vi "FastWriter.vi"() -> ()   [LabVIEW 2012]
uses:
  WVD-MCSupdate/WVDNewArchitectureUpdate/WVD_Architecture_Update/TypeDefinitions.llb/TypeDef_MPDUnitID.ctl
panel:
  out "Receive Buffer Size":u32
  out "WriteCount":i32
  out "LoopCount":i32
  out "error out":errorcluster
  in  "stop":bool
  in  "MPDUnitID":T1=enum."MPD#01"
  in  "DataBasePath":string="C:\\Users\\h2odial\\WVD-MCSupdate\\WVDNewArchitectureUpdate\\WVD_Architecture_Update\\Data\\TCSPC\\"
  in  "FileBaseNameIn":string="TCSPCFastData"
  in  "UDP Port":u16=54002
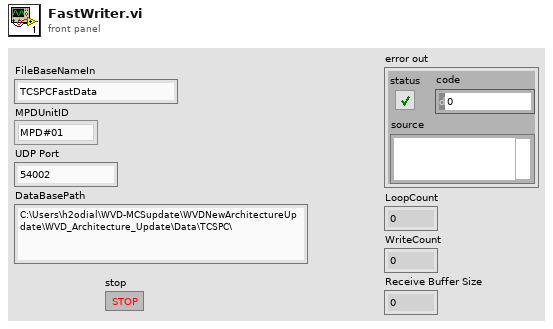
[diagram p1: front panel]
types:
  T1 = typedef "TypeDef_MPDUnitID.ctl" = enum8{"Unknown", "MPD#01", "MPD#02", "MPD#03", "MPD#04", "MPD#05"}
  T2 = enum16{"open", "replace", "create", "open or create", "replace or create", "replace or create with confirmation"}
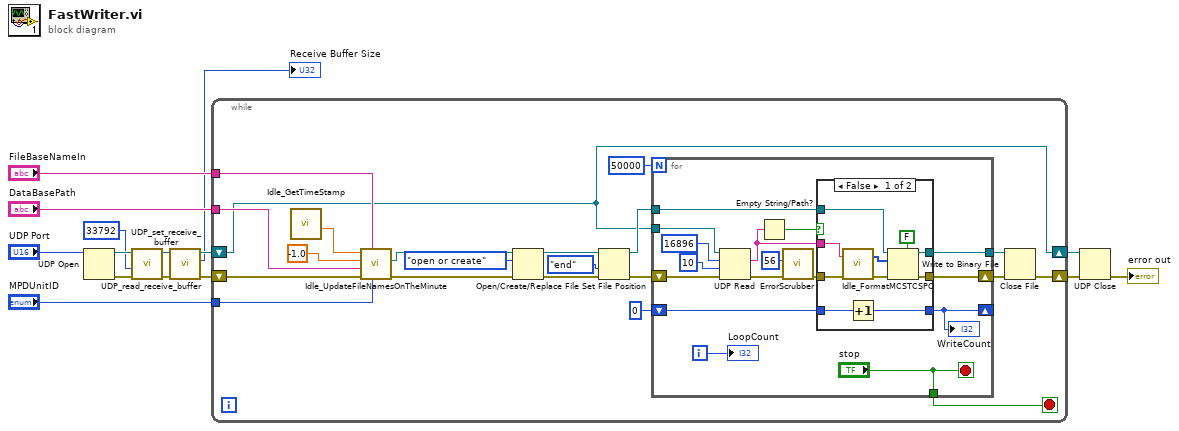
[diagram p0: block diagram]
diagram:
  n1 = UDP Open(11:"UDP Port") -> (port=w12:refnum<k16>, 0:w13:errorcluster)  [unwired: 4 in, 1 out]
  n2 = call "UDP_set_receive_buffer.vi"("error in (no error)"=w13, "Receive Buffer Size"=u32 33792, "connection ID"=w12) -> ("error out"=w10:errorcluster, "connection ID out"=w9:refnum<k16>)  [unwired: 6 in]
  n3 = call "UDP_read_receive_buffer.vi"("error in (no error)"=w10, "connection ID"=w9) -> ("error out"=w7:errorcluster, "Receive Buffer Size"=→"Receive Buffer Size":u32, "connection ID out"=w3:refnum<k16>)  [unwired: 5 in]
  n4 = while {
    shift-right: [w24] -> w15
    shift-left: w7 -> [w23]
    tunnel: "FileBaseNameIn" -> [w22]
    tunnel: "DataBasePath" -> [w21]
    tunnel: "MPDUnitID" -> [w20]
    shift-right: [w18] -> w2
    shift-left: w3 -> [w18]
    stop <- w19 stop-if-true
    n5 = call "Idle_GetTimeStamp.vi"() -> ("Fractional Hours"=w36:dbl)  [unwired: 11 in]
    n6 = call "Idle_UpdateFileNamesOnTheMinute.vi"("MPDUnitID"=w20, "FileBaseNameIn"=w22, "ErrorIn"=w23, "DataBasePathIn"=w21, "FileUpdateTimeIn"=-1.0, "CurrentTime"=w36) -> ("ErrorOur"=w30:errorcluster, "WritePathOut"=w29:path)  [unwired: 2 in, 2 out]
    n7 = Open/Create/Replace File(file path (use dialog)=w29, error in=w30, operation (0:open)=T2."open or create") -> (refnum out=w32:refnum<file>, error out=w31:errorcluster)  [unwired: 3 in, 1 out]
    n8 = Set File Position(refnum=w32, from (0:start)=enum16{"start", "end", "current"}."end", error in=w31) -> (refnum out=w28:refnum<file>, error out=w17:errorcluster)  [unwired: 1 in]
    n9 = for {
      N: 50000 -> [_]
      tunnel: w28 -> [w45]
      shift-right: [w43] -> _
      shift-left: 0 -> [w44]
      shift-right: [w41] -> w26
      shift-left: w17 -> [w42]
      tunnel: [w40] -> w25
      tunnel: w18 -> [w39]
      tunnel: ["stop"] -> w19
      i -> [w38]
      stop <- "stop" stop-if-true
      n10 = UDP Read(connection ID=w39, max size (548)=16896, timeout ms (25000)=10, 8:w42) -> (data out=w49:string, error out=w51:errorcluster)  [unwired: 3 out]
      n11 = Empty String/Path?(string/path=w49) -> (empty?=w48:bool)
      n12 = call "ErrorScrubber.vi"("error in (no error)"=w51, "y"=56) -> ("error out"=w50:errorcluster)  [unwired: 8 in, 1 out]
      n13 = case shown="False" w48 {
        tunnel: w50 -> [w62 w65]
        tunnel: w45 -> [w61 w64]
        tunnel: [w60 w64] -> w40
        tunnel: [w59 w65] -> w41
        tunnel: w49 -> [w58 _]
        tunnel: w44 -> [w57 w63]
        tunnel: [w56 w63] -> w43
        frame False {
          n14 = call "Idle_FormatMCSTCSPC.vi"("ErrorIn"=w62, "UDPResponse"=w58) -> ("ErrorOut"=w54:errorcluster, "ByteArray"=w53:u8[])
          n15 = Increment(x=w57) -> (x+1=w56:i32)
          n16 = Write to Binary File(file (use dialog)=w61, data=w53, error in=w54, 5:FALSE ("prepend array or string size? (T)")) -> (refnum out=w60:refnum<file>, error out=w59:errorcluster)  [unwired: 2 in, 1 out]
        }
        frame True {
        }
      }
      "WriteCount" <- w43
      "LoopCount" <- w38
    }
    n17 = Close File(refnum=w25, error in=w26) -> (error out=w24:errorcluster)  [unwired: 1 out]
  }
  n18 = UDP Close(connection ID=w2, 8:w15) -> (error out=→"error out":errorcluster)  [unwired: 1 out]
